vi "InitToneBuffers.vi"() -> (3 "TonesLog":T1)   [LabVIEW 2018]
doc: "Creates place holders for all of the buffer arrays for all of the tone measurements.\n(If we don't initialize these arrays, the replace array subset functions won't work.)"
uses:
  Controls/Clusts/TonesLogAll.ctl
  Controls/Clusts/ToneLogBuffered.ctl
  Controls/Enums/TargetNumber.ctl
  Controls/Clusts/SaturationMonitorBuffer.ctl
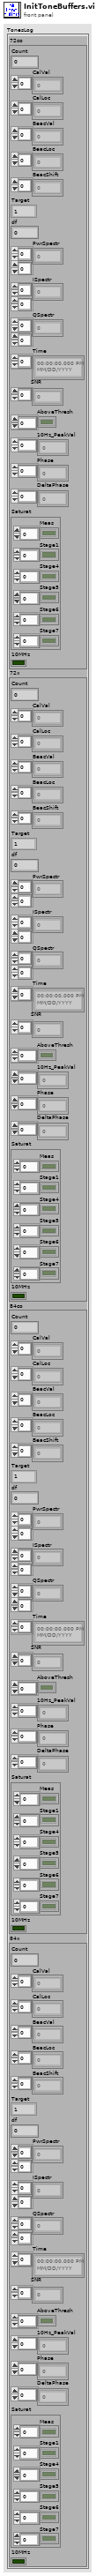
[diagram p1: front panel]
types:
  T1 = typedef "TonesLogAll.ctl" = cluster{"72co":T2, "72x":T2, "84co":T2, "84x":T2}
  T2 = typedef "ToneLogBuffered.ctl" = cluster{"Count":i32, "CalVal":sgl[], "CalLoc":i32[], "BeacVal":sgl[], "BeacLoc":i32[], "BeacShift":i32[], "Enum":T3, "df":dbl, "PwrSpectr":sgl[][], "ISpectr":sgl[][], "QSpectr":sgl[][], "Time":timestamp[], "SNR":sgl[], "AboveThresh":bool[], "10Hz_PeakVal":dbl[], "Phase":sgl[], "DeltaPhase":dbl[], "Saturat":T4, "10MHz":bool}
  T3 = typedef "TargetNumber.ctl" = enum16{"1", "2", "3", "4"}
  T4 = typedef "SaturationMonitorBuffer.ctl" = cluster{"Meas":bool[], "Stage1":bool[], "Stage4":bool[], "Stage5":bool[], "Stage6":bool[], "Stage7":bool[]}
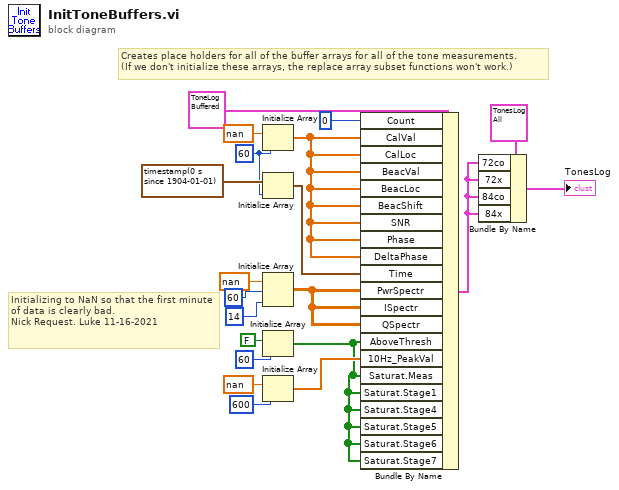
[diagram p0: block diagram]
diagram:
  w18 = 60 ("dimension size")
  # "Initializing to NaN so that the first minute of data is clearly bad.\nNick Request. Luke 11-16-2021"
  # "Creates place holders for all of the buffer arrays for all of the tone measurements.\n(If we don't initialize these arrays, the replace array subset functions won't work.)"
  n1 = Initialize Array(sgl nan ("element"), w18) -> (w1:sgl[])
  n2 = Initialize Array(timestamp(0 s since 1904-01-01), w18) -> (w19:timestamp[])
  n3 = Initialize Array(sgl nan ("Max"), 60 ("dimension size"), 14 ("dimension size")) -> (w11:sgl[][])
  n4 = Initialize Array(FALSE, 60 ("dimension size")) -> (w2:bool[])
  n5 = Initialize Array(sgl nan ("element"), 600 ("dimension size")) -> (w3:sgl[])
  n6 = Bundle By Name(cluster=T2 {"Count"=0, "CalVal"=[], "CalLoc"=[], "BeacVal"=[], "BeacLoc"=[], "BeacShift"=[], "Enum"=enum."4", "df"=0.0, "PwrSpectr"=[], "ISpectr"=[], "QSpectr"=[], "Time"=[], "SNR"=[], "AboveThresh"=[], "10Hz_PeakVal"=[], "Phase"=[], "DeltaPhase"=[], "Saturat"={"Meas"=[], "Stage1"=[], "Stage4"=[], "Stage5"=[], "Stage6"=[], "Stage7"=[]}, "10MHz"=FALSE} ("72co"), "Count"=0, "CalVal"=w1, "CalLoc"=w1, "BeacVal"=w1, "BeacLoc"=w1, "BeacShift"=w1, "SNR"=w1, "Phase"=w1, "DeltaPhase"=w1, "Time"=w19, "PwrSpectr"=w11, "ISpectr"=w11, "QSpectr"=w11, "AboveThresh"=w2, "10Hz_PeakVal"=w3, "Saturat.Meas"=w2, "Saturat.Stage1"=w2, "Saturat.Stage4"=w2, "Saturat.Stage5"=w2, "Saturat.Stage6"=w2, "Saturat.Stage7"=w2) -> (w17:T2)
  n7 = Bundle By Name(cluster=T1 {"72co"={"Count"=0, "CalVal"=[], "CalLoc"=[], "BeacVal"=[], "BeacLoc"=[], "BeacShift"=[], "Enum"=enum."4", "df"=0.0, "PwrSpectr"=[], "ISpectr"=[], "QSpectr"=[], "Time"=[], "SNR"=[], "AboveThresh"=[], "10Hz_PeakVal"=[], "Phase"=[], "DeltaPhase"=[], "Saturat"={"Meas"=[], "Stage1"=[], "Stage4"=[], "Stage5"=[], "Stage6"=[], "Stage7"=[]}, "10MHz"=FALSE}, "72x"={"Count"=0, "CalVal"=[], "CalLoc"=[], "BeacVal"=[], "BeacLoc"=[], "BeacShift"=[], "Enum"=enum."4", "df"=0.0, "PwrSpectr"=[], "ISpectr"=[], "QSpectr"=[], "Time"=[], "SNR"=[], "AboveThresh"=[], "10Hz_PeakVal"=[], "Phase"=[], "DeltaPhase"=[], "Saturat"={"Meas"=[], "Stage1"=[], "Stage4"=[], "Stage5"=[], "Stage6"=[], "Stage7"=[]}, "10MHz"=FALSE}, "84co"={"Count"=0, "CalVal"=[], "CalLoc"=[], "BeacVal"=[], "BeacLoc"=[], "BeacShift"=[], "Enum"=enum."4", "df"=0.0, "PwrSpectr"=[], "ISpectr"=[], "QSpectr"=[], "Time"=[], "SNR"=[], "AboveThresh"=[], "10Hz_PeakVal"=[], "Phase"=[], "DeltaPhase"=[], "Saturat"={"Meas"=[], "Stage1"=[], "Stage4"=[], "Stage5"=[], "Stage6"=[], "Stage7"=[]}, "10MHz"=FALSE}, "84x"={"Count"=0, "CalVal"=[], "CalLoc"=[], "BeacVal"=[], "BeacLoc"=[], "BeacShift"=[], "Enum"=enum."4", "df"=0.0, "PwrSpectr"=[], "ISpectr"=[], "QSpectr"=[], "Time"=[], "SNR"=[], "AboveThresh"=[], "10Hz_PeakVal"=[], "Phase"=[], "DeltaPhase"=[], "Saturat"={"Meas"=[], "Stage1"=[], "Stage4"=[], "Stage5"=[], "Stage6"=[], "Stage7"=[]}, "10MHz"=FALSE}} ("TonesLog"), "72co"=w17, "72x"=w17, "84co"=w17, "84x"=w17) -> (→"TonesLog":T1)
